vi "MenuDo.vi"(0 "DigitalCol in":refnum<class "DigitalCol.lvclass">, 1 "Column Array":refnum<vi>, 2 "Layout Ring Refnum":refnum<vi>, 3 "Clipboard":refnum<vi>, 5 "ItemTag":string, 7 "VariableManagerRef":refnum<vi>, 9 "Table CtlRef In":refnum<vi>, 11 "error in (no error)":errorcluster, 12 "Cell Position":T1, 13 "ModeCol Index":i32=2, 14 "Table History ref":refnum<vi>) -> (4 "DigitalCol out":refnum<class "DigitalCol.lvclass">, 6 "Col Array Ref out":refnum<vi>, 8 "Update HWI?":bool, 10 "Table CtlRef Out":refnum<vi>, 15 "error out":errorcluster)   [LabVIEW 2013, in "DigitalCol.lvclass"]
doc: "Implement shortcut menu items (added to menu by MenuBuild.vi), specific to DigitalCol. The VI starts with a parent call to catch the non-specific menu items.\nThis VI is read-only w.r.t column data."
uses:
  DigitalCol.lvclass
  <vilib>/Utility/miscctls.llb/LVRowAndColumnTypeDef.ctl
  TypeDefs/TableHistory.ctl
  TypeDefs/TableArray.ctl
  VariableManagerCodes/VariableManager/VariableManager.lvclass
  Column/Column.lvclass
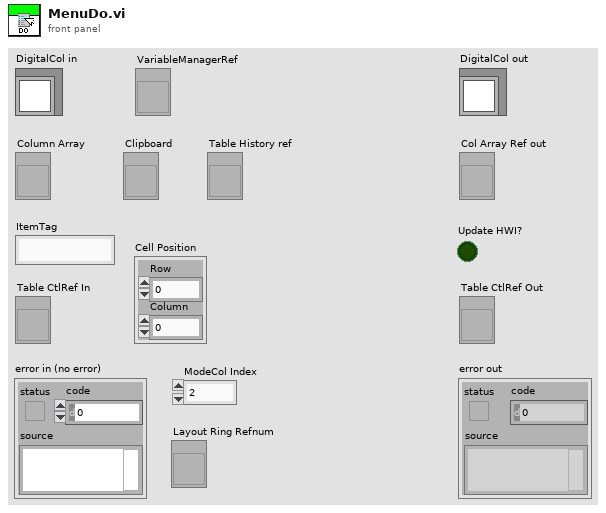
[diagram p1: front panel]
types:
  T1 = typedef "LVRowAndColumnTypeDef.ctl" = cluster{"Row":i32, "Column":i32}
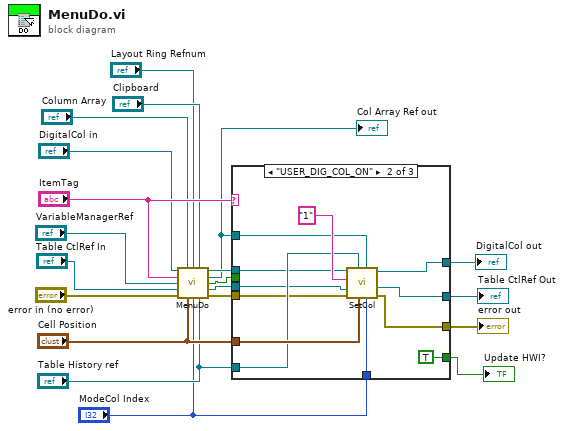
[diagram p0: block diagram]
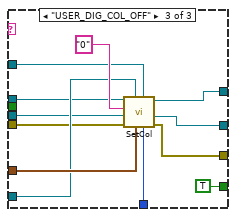
[diagram p3: hidden frame]
diagram:
  n1 = call-parent "MenuDo.vi"("Column in"="DigitalCol in", "Col Array Ref in"="Column Array", "Layout Ring Refnum"="Layout Ring Refnum", "Clipboard"="Clipboard", "ItemTag"="ItemTag", "VariableManagerRef"="VariableManagerRef", "Table CtlRef In"="Table CtlRef In", "error in (no error)"="error in (no error)", "Cell Position"="Cell Position", "ModeCol Index"="ModeCol Index", "Table History ref"="Table History ref") -> ("Column out"=w13:refnum<class "DigitalCol.lvclass">, "Col Array Ref out"=w5:refnum<vi>, "Update HWI?"=w2:bool, "Table CtlRef Out"=w11:refnum<vi>, "error out"=w12:errorcluster)
  "Col Array Ref out" <- w5
  n2 = case shown="\"USER_DIG_COL_ON\"" "ItemTag" {
    tunnel: "Cell Position" -> [_ w36 w48]
    tunnel: [w24 w35 w47] -> w20
    tunnel: [w23 w34 w46] -> w19
    tunnel: [w22 w33 w45] -> w18
    tunnel: "Table History ref" -> [_ w31 w43]
    tunnel: w13 -> [w24 w30 w42]
    tunnel: w12 -> [w22 w29 w40]
    tunnel: w11 -> [w23 w28 w41]
    tunnel: "ModeCol Index" -> [_ w27 w38]
    tunnel: w5 -> [_ w26 w39]
    tunnel: w2 -> [w21 _ _]
    tunnel: [w21 TRUE ("Update HWI?") TRUE ("Update HWI?")] -> w1
    frame Default {
    }
    frame "USER_DIG_COL_ON" {
      n3 = call-dynamic "SetCol.vi"("ModeCol Index"=w27, "Col Array Ref in"=w26, "Cell Position"=w36, "Table History ref"=w31, "error in (no error)"=w29, "Table CtlRef In"=w28, "SetTo"="1", "DigitalCol in"=w30) -> ("error out"=w33:errorcluster, "Table CtlRef Out"=w34:refnum<vi>, "DigitalCol out"=w35:refnum<class "DigitalCol.lvclass">)  [unwired: 1 out]
    }
    frame "USER_DIG_COL_OFF" {
      n4 = call-dynamic "SetCol.vi"("ModeCol Index"=w38, "Col Array Ref in"=w39, "Cell Position"=w48, "Table History ref"=w43, "error in (no error)"=w40, "Table CtlRef In"=w41, "SetTo"="0", "DigitalCol in"=w42) -> ("error out"=w45:errorcluster, "Table CtlRef Out"=w46:refnum<vi>, "DigitalCol out"=w47:refnum<class "DigitalCol.lvclass">)  [unwired: 1 out]
    }
  }
  "error out" <- w18
  "DigitalCol out" <- w20
  "Table CtlRef Out" <- w19
  "Update HWI?" <- w1
